vi "Assert String Not Contains.vi"(4 "Execution time (s)":dbl=-1.0, 5 "Assert Only? (F)":bool, 6 "error code (1)":i32=1, 7 "Label (\"\")":string, 8 "error in (no error)":errorcluster, 9 "Register with caller test (F)":bool, 10 "Substring":string, 11 "String":string) -> (0 "error out":errorcluster, 2 "Properties.Assert":refnum<class "Properties.Assert.lvclass">)   [LabVIEW 2013, in "Caraya.lvlib" / "Assert.lvclass"]
doc: "Asserts that a string does not contain a substring."
uses:
  Assert.lvclass
  Properties.Assert/Properties.Assert.lvclass
  Properties/Properties.lvclass
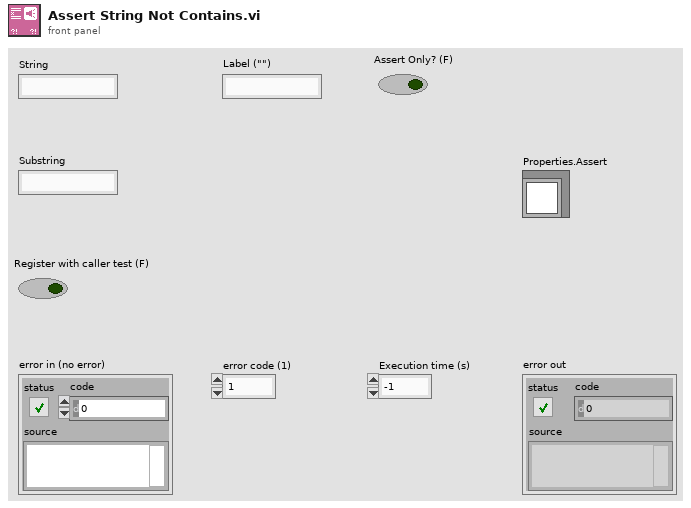
[diagram p1: front panel]
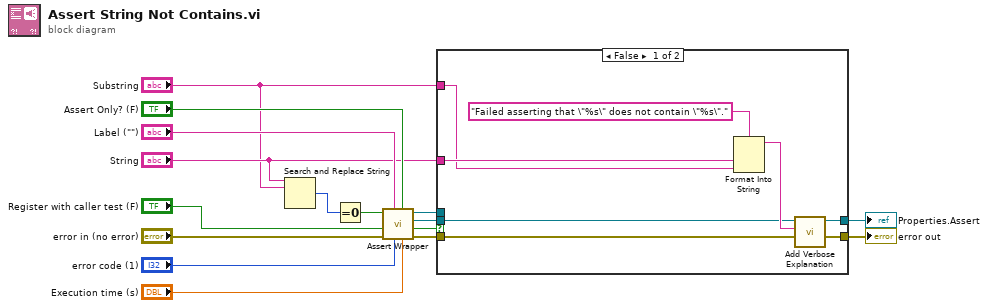
[diagram p0: block diagram]
diagram:
  n1 = Search and Replace String(input string="String", search string="Substring") -> (number of replacements=w2:i32)  [unwired: 6 in, 3 out]
  n2 = Equal To 0?(x=w2) -> (x = 0?=w1:bool)
  n3 = call "Assert Wrapper.vi"("Execution time (s)"="Execution time (s)", "Assert Only? (F)"="Assert Only? (F)", "error code (1)"="error code (1)", "Label"="Label (\"\")", "error in (no error)"="error in (no error)", "Register with caller test (F)"="Register with caller test (F)", "Assert?"=w1) -> ("error out"=w6:errorcluster, "Verbose"=w10:bool, "Properties.Assert"=w8:refnum<class "Properties.Assert.lvclass">, "Assert out"=w9:refnum<class "Assert.lvclass">)  [unwired: 1 in]
  n4 = case shown="False" w10 {
    tunnel: w9 -> [_ _]
    tunnel: w8 -> [w19 w26]
    tunnel: [w21 w25] -> w7
    tunnel: w6 -> [w22 w25]
    tunnel: "Substring" -> [w23 _]
    tunnel: "String" -> [w24 _]
    tunnel: [w18 w26] -> w5
    frame False {
      n5 = Format Into String(format string="Failed asserting that \"%s\" does not contain \"%s\".", w24, w23) -> (resulting string=w20:string)  [unwired: 2 in, 1 out]
      n6 = call "Add Verbose Explanation.vi"("error in (no error)"=w22, "Verbose Explanation"=w20, "Properties"=w19) -> ("error out"=w21:errorcluster, "Properties"=w18:refnum<class "Properties.Assert.lvclass">)  [unwired: 7 in]
    }
    frame True {
    }
  }
  "error out" <- w7
  "Properties.Assert" <- w5
